vi "HH coils on off - BK9129B.VI"(9 "BKcoil VISA":refnum<visa-resource-name>="BK9123A_moe", 11 "coils on?":bool=TRUE) -> ()   [LabVIEW 2020]
panel:
  in  "Serial Configuration":T1={"Parity(0:none)"=0, "Baud Rate (9600)"=9600, "Data Bits(8)"=8, "Flow Control(None)"=0, " Stop Bits(1.0)"=10} {"Stop Bits(1.0)" items=["1.0"=10, "1.5"=15, "2.0"=20]; "Flow Control(None)" items=["None", "XON/XOFF", "RTS/CTS", "XON/XOFF & RTS/CTS", "DTR/DSR", "XON/XOFF & DTR/DSR"]; "Data Bits(8)" items=["7"=7, "8"=8]; "Baud Rate (9600)" items=["2400"=2400, "4800"=4800, "9600"=9600, "19200"=19200, "38400"=38400]; "Parity(0:none)" items=["None", "Odd", "Even", "Mark", "Space"]}
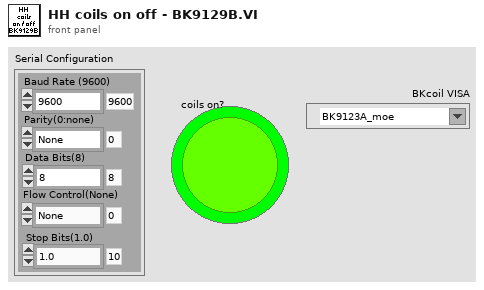
[diagram p1: front panel]
types:
  T1 = cluster{"Parity(0:none)":u16, "Baud Rate (9600)":u16, "Data Bits(8)":u16, "Flow Control(None)":u16, " Stop Bits(1.0)":u16}
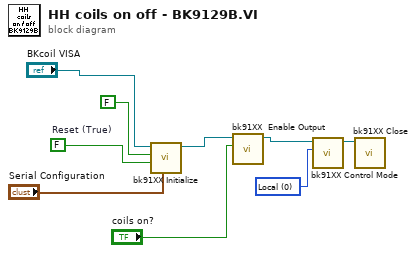
[diagram p0: block diagram]
diagram:
  w4 = FALSE items=["OFF", "ON", "OFF", "ON"]  # Reset (True)
  w7 = u16 0 items=["Local", "Remote"] ("Control Mode(1:Remote)")
  n1 = call "bk91XX Initialize.vi"("Serial Configuration"="Serial Configuration", "Reset (True)"=w4, "ID Query (True)"=FALSE, "VISA resource name"="BKcoil VISA") -> ("VISA resource name out"=w1:refnum<visa-resource-name>)  [unwired: 6 in, 1 out]
  n2 = call "bk91XX  Enable Output.vi"("Enable Output (T: Enable)"="coils on?", "VISA resource name"=w1) -> ("VISA resource name out"=w6:refnum<visa-resource-name>)  [unwired: 8 in, 1 out]
  n3 = call "bk91XX Control Mode.vi"("Control Mode (1: Remote)"=w7, "VISA resource name"=w6) -> ("VISA resource name out"=w8:refnum<visa-resource-name>)  [unwired: 8 in, 1 out]
  n4 = call "bk91XX Close.vi"("VISA resource name"=w8) -> ()  [unwired: 10 in, 1 out]
